vi "loadFileNewFindOutCounter.vi"(10 "folder":string="QAMT01\\CRH3605", 11 "Entity":string) -> (1 "f":bool, 3 "Lot":string)   [LabVIEW 2012]
uses:
  Global1.vi
panel:
  out "error out":errorcluster
  in  "error in (no error)":errorcluster
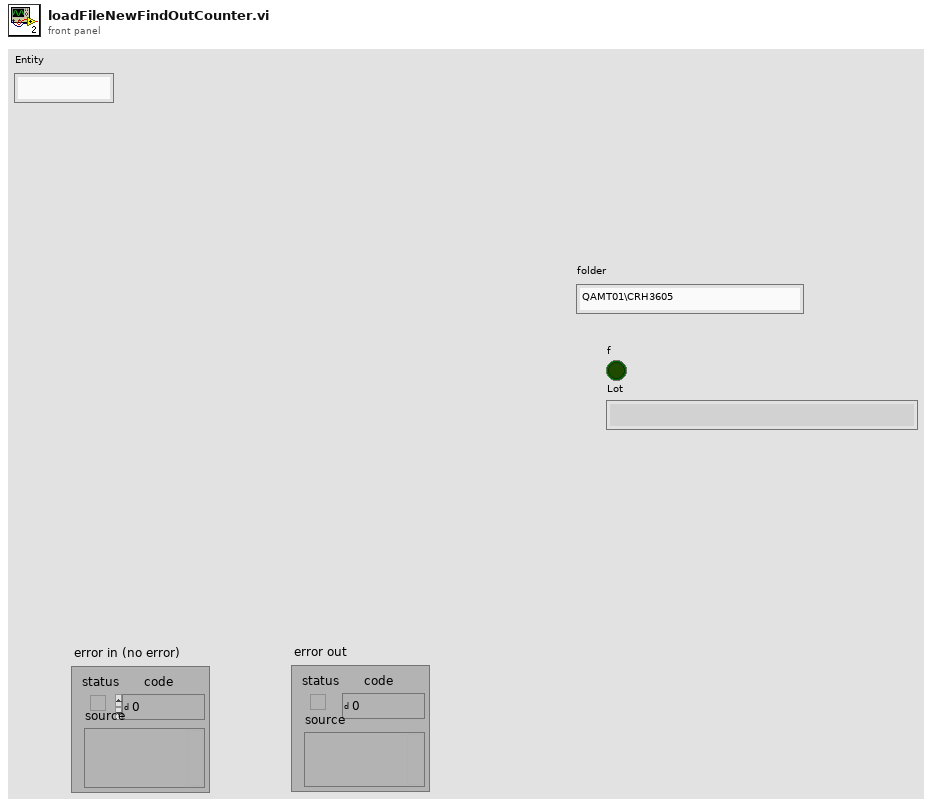
[diagram p1: front panel]
types:
  T1 = enum16{"open", "replace", "create", "open or create", "replace or create", "replace or create with confirmation"}
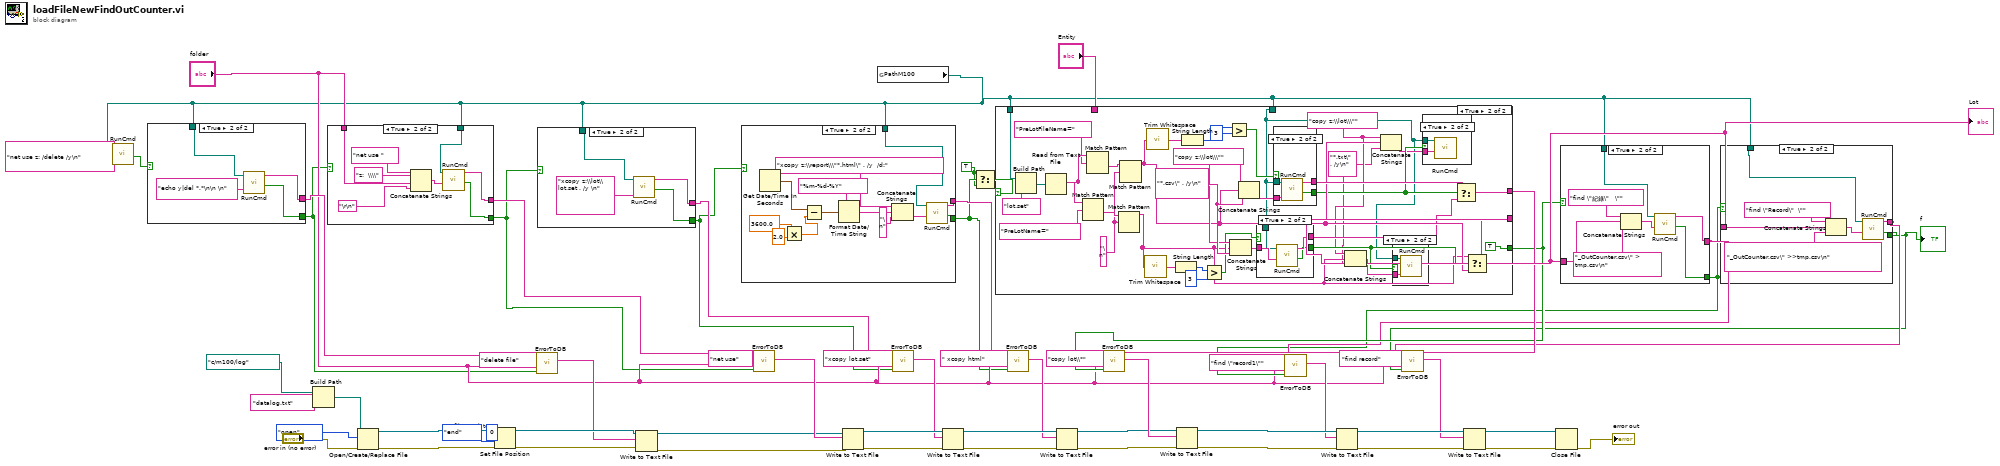
[diagram p0: block diagram]
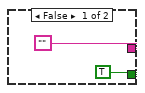
[diagram p2: hidden frame]
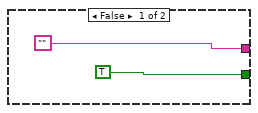
[diagram p3: hidden frame]
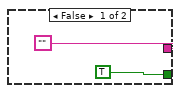
[diagram p4: hidden frame]
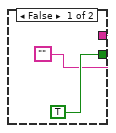
[diagram p5: hidden frame]
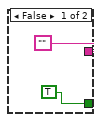
[diagram p6: hidden frame]
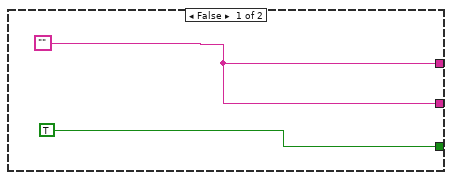
[diagram p7: hidden frame]
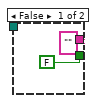
[diagram p10: hidden frame]
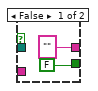
[diagram p11: hidden frame]
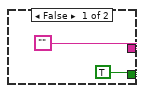
[diagram p12: hidden frame]
diagram:
  w8 = TRUE
  # "Set file mark to\nend of file"
  n1 = Build Path(base path=path "c:/m100/log", name or relative path="datalog.txt") -> (appended path=w54:path)
  n2 = Open/Create/Replace File(file path (use dialog)=w54, error in="error in (no error)", operation (0:open)=T1."open") -> (refnum out=w59:refnum<file>, error out=w58:errorcluster)  [unwired: 3 in, 1 out]
  n3 = Set File Position(offset (in bytes) (0)=i64 0, refnum=w59, from (0:start)=enum16{"start", "end", "current"}."end", error in=w58) -> (refnum out=w24:refnum<file>, error out=w23:errorcluster)
  n4 = global read "Global1.vi" "PathM100"() -> (w1:path)
  n5 = call "RunCmd.vi"("Cmd String"="net use z: /delete /y\n" ("string"), "working directory"=w1) -> ("OK"=w25:bool)  [unwired: 8 in, 1 out]
  n6 = case shown="True" w25 {
    tunnel: [TRUE w66] -> w6
    tunnel: ["" w65] -> w20
    tunnel: w1 -> [_ w68]
    frame False {
    }
    frame True {
      n7 = call "RunCmd.vi"("Cmd String"="echo y|del *.*\n\n \n" ("standard input"), "working directory"=w68) -> ("OK"=w66:bool, "Output"=w65:string)  [unwired: 8 in]
    }
  }
  n8 = case shown="True" w6 {
    tunnel: [TRUE w71] -> w7
    tunnel: ["" w72] -> w33
    tunnel: "folder" -> [_ w74]
    tunnel: w1 -> [_ w73]
    frame False {
    }
    frame True {
      n9 = Concatenate Strings("net use " ("string"), "z:  \\\\" ("string"), w74, "\r\n") -> (w78:string)
      n10 = call "RunCmd.vi"("Cmd String"=w78, "working directory"=w73) -> ("OK"=w71:bool, "Output"=w72:string)  [unwired: 8 in]
    }
  }
  n11 = call "ErrorToDB.vi"("Error"=w6, "Folder"="folder", "Command"="delete file", "Error Message"=w20) -> ("LogData"=w19:string)  [unwired: 7 in]
  n12 = case shown="True" w7 {
    tunnel: [TRUE w82] -> w5
    tunnel: ["" w81] -> w32
    tunnel: w1 -> [_ w84]
    frame False {
    }
    frame True {
      n13 = call "RunCmd.vi"("Cmd String"="xcopy z:\\lot\\lot.set . /y \n" ("standard input"), "working directory"=w84) -> ("OK"=w82:bool, "Output"=w81:string)  [unwired: 8 in]
    }
  }
  n14 = Write to Text File(file (use dialog)=w24, text=w19, error in=w23) -> (refnum out=w22:refnum<file>, error out=w21:errorcluster)  [unwired: 1 in, 1 out]
  n15 = case shown="True" w5 {
    tunnel: [TRUE w88] -> w10
    tunnel: ["" w89] -> w31
    tunnel: w1 -> [_ w87]
    frame False {
    }
    frame True {
      n16 = Get Date/Time In Seconds() -> (seconds since 1Jan1904=w90:timestamp)
      n17 = Multiply(x=3600.0, y=2.0) -> (x*y=w92:dbl)
      n18 = Subtract(x=w90, y=w92) -> (x-y=w93:timestamp)
      n19 = Format Date/Time String(time format string (%c)="%m-%d-%Y", seconds (now)=w93) -> (date/time string=w96:string)  [unwired: 1 in]
      n20 = Concatenate Strings("xcopy z:\\report\\\"*.html\" . /y  /d:" ("string"), w96, "\n" ("string")) -> (w99:string)
      n21 = call "RunCmd.vi"("Cmd String"=w99, "working directory"=w87) -> ("OK"=w88:bool, "Output"=w89:string)  [unwired: 8 in]
    }
  }
  n22 = call "ErrorToDB.vi"("Error"=w7, "Folder"="folder", "Command"="net use", "Error Message"=w33) -> ("LogData"=w44:string)  [unwired: 7 in]
  n23 = Write to Text File(file (use dialog)=w22, text=w44, error in=w21) -> (refnum out=w53:refnum<file>, error out=w52:errorcluster)  [unwired: 1 in, 1 out]
  n24 = call "ErrorToDB.vi"("Error"=w5, "Folder"="folder", "Command"="xcopy lot.set", "Error Message"=w32) -> ("LogData"=w43:string)  [unwired: 7 in]
  n25 = Write to Text File(file (use dialog)=w53, text=w43, error in=w52) -> (refnum out=w30:refnum<file>, error out=w29:errorcluster)  [unwired: 1 in, 1 out]
  n26 = Select(t=w8, s=w10, f=w8) -> (s? t:f=w9:bool)
  n27 = case shown="True" w9 {
    tunnel: [TRUE TRUE] -> w39
    tunnel: [w100 w121] -> w40
    tunnel: w1 -> [_ w132]
    tunnel: [w100 w122] -> w45
    tunnel: w1 -> [_ w106]
    tunnel: "Entity" -> [_ _]
    frame False {
      w100 = ""
    }
    frame True {
      w103 = "*.txt\" . /y\n" ("string")
      w105 = "copy z:\\lot\\\"" ("string")
      w127 = "\n" ("regular expression")
      w116 = "copy z:\\lot\\\"" ("string")
      w126 = "*.csv\" . /y\n" ("string")
      n28 = Build Path(base path=w132, name or relative path="lot.set") -> (appended path=w136:path)
      n29 = Read from Text File(file (use dialog)=w136) -> (text=w130:string)  [unwired: 3 in, 3 out]
      n30 = Match Pattern(string=w130, regular expression="PreLotName=") -> (after substring=w133:string)  [unwired: 1 in, 3 out]
      n31 = Match Pattern(string=w130, regular expression="PreLotFileName=") -> (after substring=w128:string)  [unwired: 1 in, 3 out]
      n32 = Match Pattern(string=w133, regular expression=w127) -> (before substring=w104:string)  [unwired: 1 in, 3 out]
      n33 = Match Pattern(string=w128, regular expression=w127) -> (before substring=w111:string)  [unwired: 1 in, 3 out]
      n34 = call <vilib>:"Trim Whitespace.vi"("string"=w104) -> ("trimmed string"=w119:string)  [unwired: 1 in]
      n35 = call <vilib>:"Trim Whitespace.vi"("string"=w111) -> ("trimmed string"=w120:string)  [unwired: 1 in]
      n36 = String Length(string=w119) -> (length=w118:i32)
      n37 = String Length(string=w120) -> (length=w115:i32)
      n38 = Greater?(x=w118, y=3) -> (0:w112:bool)
      n39 = Greater?(x=w115, y=3) -> (0:w113:bool)
      n40 = Concatenate Strings(w116, w104, w126) -> (w125:string)
      n41 = Concatenate Strings(w116, w111, w126) -> (w131:string)
      n42 = case shown="True" w112 {
        tunnel: w125 -> [_ w146]
        tunnel: w106 -> [_ w145]
        tunnel: ["" ("Output") w144] -> w107
        tunnel: [FALSE ("OK") w143] -> w108
        frame False {
        }
        frame True {
          n43 = call "RunCmd.vi"("Cmd String"=w146, "working directory"=w145) -> ("OK"=w143:bool, "Output"=w144:string)  [unwired: 8 in]
        }
      }
      n44 = case shown="True" w113 {
        tunnel: w131 -> [_ w152]
        tunnel: w106 -> [_ w151]
        tunnel: [FALSE ("OK") w150] -> w110
        tunnel: ["" ("Output") w149] -> w124
        frame False {
        }
        frame True {
          n45 = call "RunCmd.vi"("Cmd String"=w152, "working directory"=w151) -> ("OK"=w150:bool, "Output"=w149:string)  [unwired: 8 in]
        }
      }
      n46 = Concatenate Strings(w105, w104, w103) -> (w102:string)
      n47 = Concatenate Strings(w105, w111, w103) -> (w109:string)
      n48 = case shown="True" w108 {
        tunnel: w106 -> [_ w138]
        tunnel: w102 -> [_ w137]
        frame False {
        }
        frame True {
          n49 = call "RunCmd.vi"("Cmd String"=w137, "working directory"=w138) -> ()  [unwired: 8 in, 2 out]
        }
      }
      n50 = case shown="True" w110 {
        tunnel: w106 -> [_ w140]
        tunnel: w109 -> [_ w139]
        frame False {
        }
        frame True {
          n51 = call "RunCmd.vi"("Cmd String"=w139, "working directory"=w140) -> ()  [unwired: 8 in, 2 out]
        }
      }
      n52 = Select(t=w124, s=w110, f=w107) -> (s? t:f=w121:string)
      n53 = Select(t=w104, s=w108, f=w111) -> (s? t:f=w122:string)
    }
  }
  "Lot" <- w45
  n54 = call "ErrorToDB.vi"("Error"=w10, "Folder"="folder", "Command"=" xcopy html", "Error Message"=w31) -> ("LogData"=w26:string)  [unwired: 7 in]
  n55 = Write to Text File(file (use dialog)=w30, text=w26, error in=w29) -> (refnum out=w28:refnum<file>, error out=w27:errorcluster)  [unwired: 1 in, 1 out]
  n56 = call "ErrorToDB.vi"("Error"=w39, "Folder"="folder", "Command"="copy lot\\*", "Error Message"=w40) -> ("LogData"=w41:string)  [unwired: 7 in]
  n57 = Write to Text File(file (use dialog)=w28, text=w41, error in=w27) -> (refnum out=w51:refnum<file>, error out=w50:errorcluster)  [unwired: 1 in, 1 out]
  n58 = case shown="True" w39 {
    tunnel: ["" w156] -> w37
    tunnel: w45 -> [_ w160]
    tunnel: w1 -> [_ w157]
    tunnel: [TRUE w155] -> w36
    frame False {
    }
    frame True {
      n59 = Concatenate Strings("find \"紀錄\"   \"" ("string"), w160, "_OutCounter.csv\" > tmp.csv\n" ("string")) -> (w158:string)
      n60 = call "RunCmd.vi"("Cmd String"=w158, "working directory"=w157) -> ("OK"=w155:bool, "Output"=w156:string)  [unwired: 8 in]
    }
  }
  n61 = call "ErrorToDB.vi"("Error"=w36, "Folder"="folder", "Command"="find \"record1\"", "Error Message"=w37) -> ("LogData"=w38:string)  [unwired: 7 in]
  n62 = Write to Text File(file (use dialog)=w51, text=w38, error in=w50) -> (refnum out=w49:refnum<file>, error out=w47:errorcluster)  [unwired: 1 in, 1 out]
  n63 = case shown="True" w36 {
    tunnel: w1 -> [_ w167]
    tunnel: w45 -> [_ w168]
    tunnel: ["" w164] -> w34
    tunnel: [TRUE w165] -> w2
    frame False {
    }
    frame True {
      n64 = Concatenate Strings("find \"Record\"  \"" ("string"), w168, "_OutCounter.csv\" >>tmp.csv\n" ("string")) -> (w166:string)
      n65 = call "RunCmd.vi"("Cmd String"=w166, "working directory"=w167) -> ("OK"=w165:bool, "Output"=w164:string)  [unwired: 8 in]
    }
  }
  "f" <- w2
  n66 = call "ErrorToDB.vi"("Error"=w2, "Folder"="folder", "Command"="find record", "Error Message"=w34) -> ("LogData"=w35:string)  [unwired: 7 in]
  n67 = Write to Text File(file (use dialog)=w49, text=w35, error in=w47) -> (refnum out=w48:refnum<file>, error out=w46:errorcluster)  [unwired: 1 in, 1 out]
  n68 = Close File(refnum=w48, error in=w46) -> (error out=→"error out":errorcluster)  [unwired: 1 out]
